vi "QT_QTImageToLVPict+.vi"(1 "Draw info":bool=TRUE, 2 "Image/Movie Out":T2={"Width"=160, "Height"=120, "Depth"=32, "data"=array[76800 elements], "Compressed data"=array[6408 elements], "Color table"=[], "Duration"=0, "Options"=0, "Timestamp"=0, "ID"=265, "Reserved"=0, "Dialogs"=0} {"Dialogs" format="%.0b"}, 3 "BW image":bool, 5 "Thresholds":T1 {"Blue threshold" format="%.2f"; "Green threshold" format="%.2f"; "Red threshold" format="%.2f"; "BW threshold" format="%.2f"}) -> (9 "Timestamp":i32, 13 "ID":i32=265, 14 "Picture color":picture, 15 "Picture B&W/Alpha channel":picture, 16 "R":picture, 17 "G":picture, 18 "B":picture, 19 "Pict Draw Area Size":cluster{"Width":i16, "Height":i16}={"Width"=160, "Height"=120})   [LabVIEW 2024]
uses:
  <userlib>/ImageProcessing/QTLIB_2595_LV86/QT_Image.ctl
  <userlib>/ImageProcessing/QTLIB_2595_LV86/QT_Thresholds.ctl
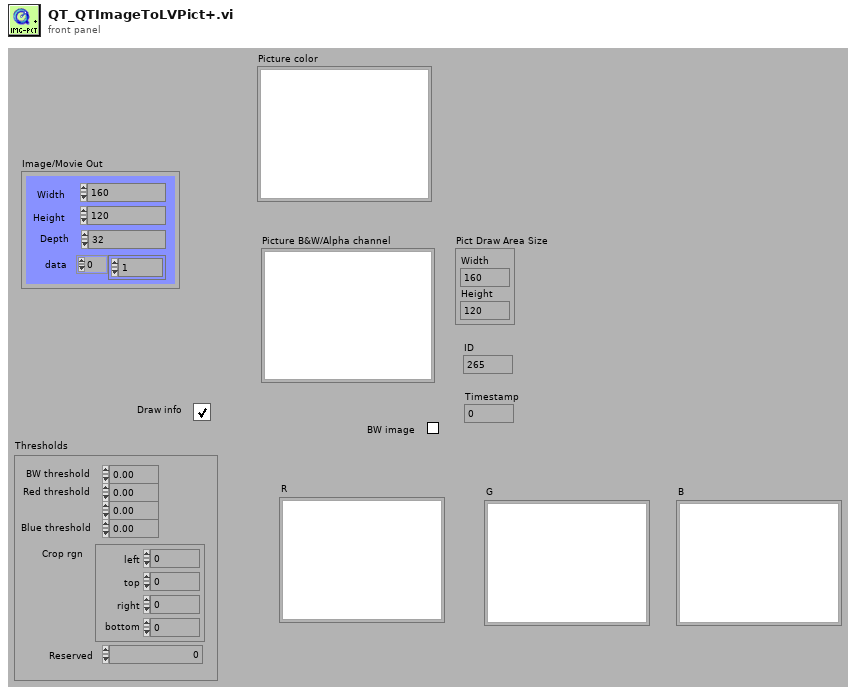
[diagram p1: front panel]
types:
  T1 = typedef "QT_Thresholds.ctl" = cluster{"BW threshold":dbl, "Red threshold":dbl, "Green threshold":dbl, "Blue threshold":dbl, "Crop rgn":cluster{"left":i16, "top":i16, "right":i16, "bottom":i16}, "Reserved":i32}
  T2 = typedef "QT_Image.ctl" = cluster{"Width":i32, "Height":i32, "Depth":i32, "data":u8[], "Compressed data":u8[], "Color table":u32[], "Duration":i32, "Options":i32, "Timestamp":i32, "ID":i32, "Reserved":i32, "Dialogs":u32}
  T3 = cluster{"left":i16, "top":i16, "right":i16, "bottom":i16}
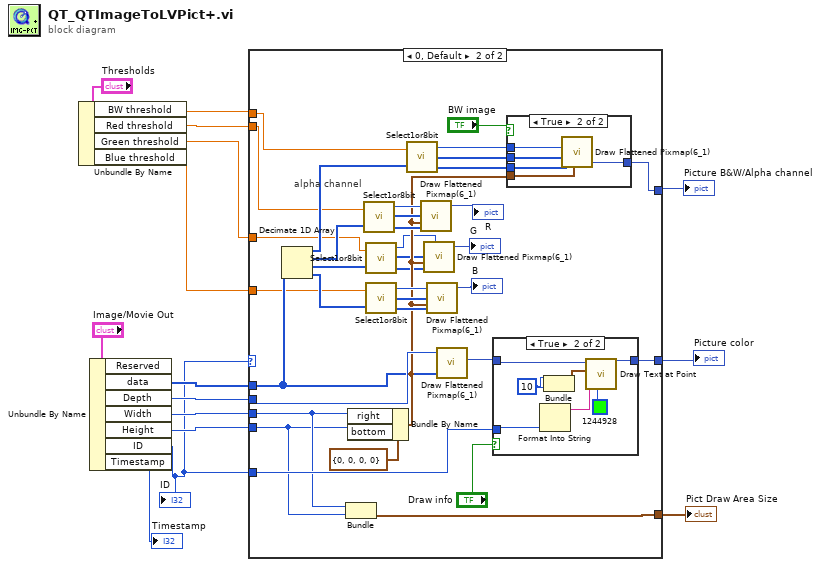
[diagram p0: block diagram]
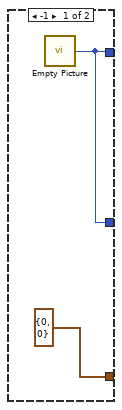
[diagram p2: hidden frame]
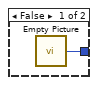
[diagram p3: hidden frame]
diagram:
  n1 = Unbundle By Name("Thresholds") -> ("BW threshold"=w4:dbl, "Red threshold"=w3:dbl, "Green threshold"=w2:dbl, "Blue threshold"=w1:dbl)
  n2 = Unbundle By Name("Image/Movie Out") -> ("data"=w15:u8[], "Depth"=w13:i32, "Width"=w12:i32, "Height"=w11:i32, "ID"=w8:i32, "Timestamp"=→"Timestamp":i32)  [unwired: 1 out]
  "ID" <- w8
  n3 = case shown="0, Default" w8 {
    tunnel: w15 -> [_ w43]
    tunnel: w13 -> [_ w44]
    tunnel: w12 -> [_ w46]
    tunnel: w11 -> [_ w45]
    tunnel: [w17 w53] -> w10
    tunnel: [w17 w52] -> w9
    tunnel: w8 -> [_ w51]
    tunnel: [cluster{"Width":i16, "Height":i16} {"Width"=0, "Height"=0} ("Pict Draw Area Size") w47] -> w7
    tunnel: w4 -> [_ w37]
    tunnel: w3 -> [_ w35]
    tunnel: w2 -> [_ w32]
    tunnel: w1 -> [_ w31]
    frame -1 {
      n4 = call "Empty Picture"() -> ("empty picture"=w17:picture)
    }
    frame 0, Default {
      # "alpha channel"
      n5 = Decimate 1D Array(w43) -> (w40:u8[], w36:u8[], w34:u8[], w33:u8[])
      n6 = Bundle("Width"=w46, "Height"=w45) -> (w47:cluster{"Width":i32, "Height":i32})  [unwired: 1 out]
      n7 = Bundle By Name(cluster=T3 {"left"=0, "top"=0, "right"=0, "bottom"=0} ("rect"), "right"=w46, "bottom"=w45) -> (w23:T3)
      n8 = call <userlib>:"Select1or8bit.vi"("BW threshold"=w35, "Array 2"=w36) -> ("bit depth(8)"=w29:u8, "Color Table"=w28:u32[], "[packed (8) booleans] as [u8]"=w30:u8[])
      n9 = call <userlib>:"Select1or8bit.vi"("BW threshold"=w32, "Array 2"=w34) -> ("bit depth(8)"=w20:u8, "Color Table"=w21:u32[], "[packed (8) booleans] as [u8]"=w22:u8[])
      n10 = call <userlib>:"Select1or8bit.vi"("BW threshold"=w31, "Array 2"=w33) -> ("bit depth(8)"=w24:u8, "Color Table"=w25:u32[], "[packed (8) booleans] as [u8]"=w26:u8[])
      n11 = call <userlib>:"Select1or8bit.vi"("BW threshold"=w37, "Array 2"=w40) -> ("bit depth(8)"=w42:u8, "Color Table"=w38:u32[], "[packed (8) booleans] as [u8]"=w39:u8[])
      n12 = call <vilib>:"Draw Flattened Pixmap(6_1).vi"("bit depth(8)"=w29, "rect"=w23, "flattened pixmap data"=w30, "color table"=w28) -> ("new picture"=→"R":picture)  [unwired: 1 in, 4 out]
      n13 = call <vilib>:"Draw Flattened Pixmap(6_1).vi"("bit depth(8)"=w20, "rect"=w23, "flattened pixmap data"=w22, "color table"=w21) -> ("new picture"=→"G":picture)  [unwired: 1 in, 4 out]
      n14 = call <vilib>:"Draw Flattened Pixmap(6_1).vi"("bit depth(8)"=w24, "rect"=w23, "flattened pixmap data"=w26, "color table"=w25) -> ("new picture"=→"B":picture)  [unwired: 1 in, 4 out]
      n15 = call <vilib>:"Draw Flattened Pixmap(6_1).vi"("bit depth(8)"=w44, "rect"=w23, "flattened pixmap data"=w43) -> ("new picture"=w41:picture)  [unwired: 2 in, 4 out]
      n16 = case shown="True" "Draw info" {
        tunnel: w41 -> [w60 w67]
        tunnel: [w60 w66] -> w52
        tunnel: w51 -> [_ w62]
        frame False {
        }
        frame True {
          w63 = i16 10 ("left")
          n17 = Format Into String(w62) -> (resulting string=w61:string)  [unwired: 3 in, 1 out]
          n18 = Bundle("left"=w63, "left"=w63) -> (w65:cluster{"left":i16, "left":i16})  [unwired: 1 out]
          n19 = call <vilib>:"Draw Text at Point.vi"("text color(black)"=u32 1244928, "text"=w61, "origin"=w65, "picture"=w67) -> ("new picture"=w66:picture)  [unwired: 5 in, 2 out]
        }
      }
      n20 = case shown="True" "BW image" {
        tunnel: w39 -> [_ w59]
        tunnel: w23 -> [_ w58]
        tunnel: [w54 w57] -> w53
        tunnel: w42 -> [_ w56]
        tunnel: w38 -> [_ w55]
        frame False {
          n21 = call "Empty Picture"() -> ("empty picture"=w54:picture)
        }
        frame True {
          n22 = call <vilib>:"Draw Flattened Pixmap(6_1).vi"("bit depth(8)"=w56, "rect"=w58, "flattened pixmap data"=w59, "color table"=w55) -> ("new picture"=w57:picture)  [unwired: 1 in, 4 out]
        }
      }
    }
  }
  "Picture color" <- w9
  "Picture B&W/Alpha channel" <- w10
  "Pict Draw Area Size" <- w7
